vi "Teleop.vi"(10 "Match Info":T1={"Autonomous Elapsed Seconds"=0.0, "TeleOp Elapsed Seconds"=0.0, "Disabled Elapsed Seconds"=0.0, "Visited Autonomous"=FALSE, "Visited TeleOp"=FALSE, "Visited Disabled"=FALSE, "Autonomous Settings"={"Autonomous Style"=enum."Independent", "VI Refnum"=refnum}}, 11 "Call Context":T2) -> ()   [LabVIEW 2012]
doc: "This VI is called for each TeleOp packet received from the DS where the robot is not disabled. It is often used to read from the joysticks and update I/O or to update setpoints for timed control loops. It should complete and return within 20 milliseconds or it may miss DS packets."
uses:
  <vilib>/Rock Robotics/WPI/DriverStation/WPI_DriverStationDerivedRobotMode.ctl
  <vilib>/Rock Robotics/WPI/DriverStation/WPI_DriverStationMatch Info.ctl
  Robot Global Data.vi
  BotStatus.vi
  <vilib>/Rock Robotics/WPI/Joystick/WPI_JoystickGetSetRefNum.vi
  <vilib>/Rock Robotics/WPI/RobotDrive/WPI_RobotDriveGetSetRefNum.vi
panel:
  out "Numeric 1":dbl(slide) scale=0.0..100.0
  out "Boolean 2":bool
  out "Boolean 1":bool
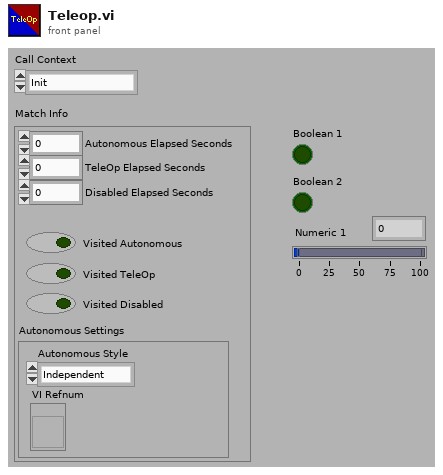
[diagram p1: front panel]
types:
  T1 = typedef "WPI_DriverStationMatch Info.ctl" = cluster{"Autonomous Elapsed Seconds":dbl, "TeleOp Elapsed Seconds":dbl, "Disabled Elapsed Seconds":dbl, "Visited Autonomous":bool, "Visited TeleOp":bool, "Visited Disabled":bool, "Autonomous Settings":cluster{"Autonomous Style":enum16{"Iterative", "Independent"}, "VI Refnum":refnum<vi>}}
  T2 = typedef "WPI_DriverStationDerivedRobotMode.ctl" = enum16{"Init", "Execute", "Stop"}
  T3 = typedef "WPI_JoystickDevRef.ctl" = cluster{"Device":T4}
  T4 = typedef "WPI_JoystickDeviceEnum.ctl" = enum16{"USB 1", "USB 2", "USB 3", "USB 4", "Kinect 1", "Kinect 2"}
  T5 = cluster{"Target Position X":dbl, "Target Position Y":dbl, "Target Found":bool}
  T6 = typedef "WPI_ServoDeviceRef.ctl" = cluster{"DeviceStatus":errorcluster, "Digital Module":T7, "PWM Channel":T8, "DeadBand":T9}
  T7 = typedef "FPGA_TypedefDigitalModule.ctl" = enum16{"Digital Module 1", "Digital Module 2"}
  T8 = typedef "FPGA_DIOPWMChannel.ctl" = enum8{"PWM 1", "PWM 2", "PWM 3", "PWM 4", "PWM 5", "PWM 6", "PWM 7", "PWM 8", "PWM 9", "PWM 10", "Invalid"}
  T9 = typedef "WPI_PWMDeadband.ctl" = cluster{"Name":string, "maxPositivePwm":i32, "minPositivePwm":i32, "centerPwm":i32, "maxNegativePwm":i32, "minNegativePwm":i32, "angularRange":u16}
  T10 = typedef "WPI_RobotDriveDevRef.ctl" = cluster{"DevStatus":errorcluster, "Motors[]":T11[], "Square Inputs":bool, "Max Output":dbl, "Isochronous":bool}
  T11 = typedef "WPI_MotorControlDeviceRef.ctl" = cluster{"DeviceStatus":errorcluster, "Type":enum16{"PWM", "CAN"}, "PWM":cluster{"Digital Module":T7, "PWM Channel":T8, "DeadBand":T9}, "CAN":cluster{"Device Number":u8, "Control Mode":T12, "Semaphore":T13, "Max Vout":dbl}, "Invert":bool, "TransformRef":T14, "InvTransformRef":T14}
  T12 = typedef "WPI_CANJaguar_ControlMode.ctl" = enum8{"Percent VBus", "Current", "Speed", "Position", "Voltage"}
  T13 = typedef "Semaphore RefNum" = refnum<k1>
  T14 = typedef "WPI_PWMTransform_ConPane.ctl" = refnum<vi>
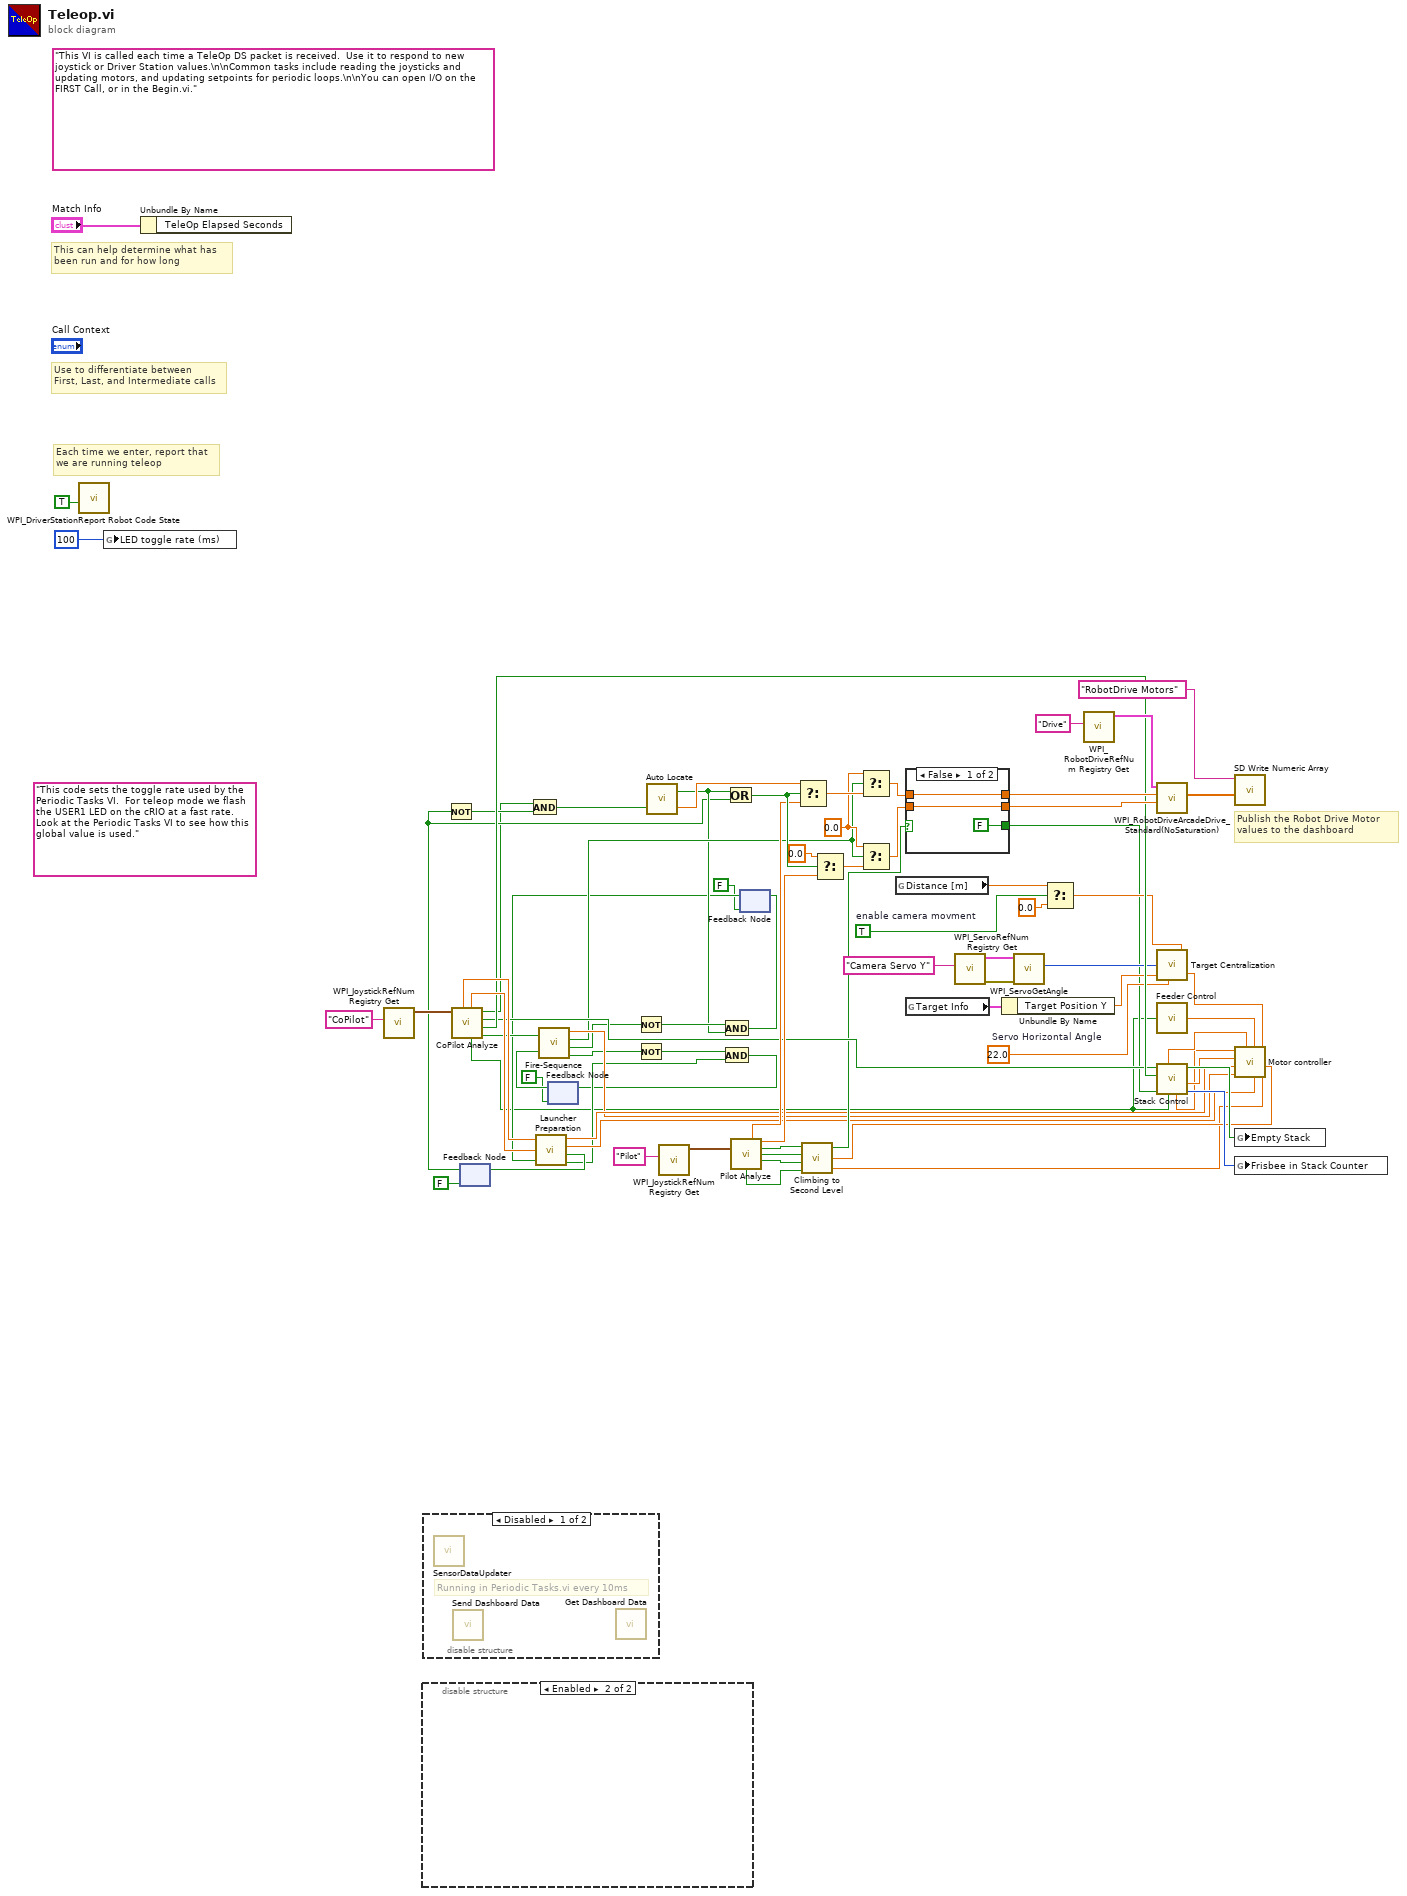
[diagram p0: block diagram]
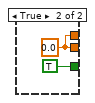
[diagram p3: hidden frame]
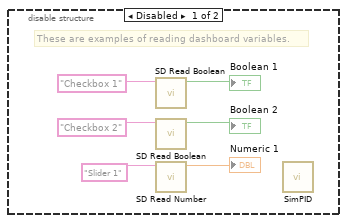
[diagram p4: hidden frame]
diagram:
  w32 = 22.0  # Servo Horizontal Angle
  w38 = TRUE  # enable camera movment
  w59 = 0.0
  (unwired) "This code sets the toggle rate used by the Periodic Tasks VI.  For teleop mode we flash the USER1 LED on the cRIO at a fast rate.  Look at the Periodic Tasks VI to see how this global value is used."
  (unwired) "This VI is called each time a TeleOp DS packet is received.  Use it to respond to new joystick or Driver Station values.\n\nCommon tasks include reading the joysticks and updating motors, and updating setpoints for periodic loops.\n\nYou can open I/O on the FIRST Call, or in the Begin.vi."
  # "Publish the Robot Drive Motor\nvalues to the dashboard"
  # "Each time we enter, report that\nwe are running teleop"
  # "Use to differentiate between\nFirst, Last, and Intermediate calls"
  # "This can help determine what has\nbeen run and for how long"
  n1 = call <vilib>:"WPI_DriverStationReport Robot Code State.vi"("TeleOp"=TRUE ("Autonomous")) -> ()  [unwired: 10 in, 1 out]
  n2 = global write "Robot Global Data.vi" "LED toggle rate (ms)"(u32 100 ("LED ms toggle rate")) -> ()
  n3 = Unbundle By Name("Match Info") -> ()  [unwired: 1 out]
  n4 = call <vilib>:"WPI_JoystickRefNum Registry Get.vi"("refnum name"="CoPilot") -> ("JoystickDevRef"=w67:T3)  [unwired: 1 in, 9 out]
  n5 = disable-structure shown="Enabled" {
    frame Disabled {
      # "These are examples of reading dashboard variables."
      n6 = call <vilib>:"SD Read Boolean.vi"("Name"="Checkbox 1" ("refnum name")) -> ("Boolean"=→"Boolean 1":bool)  [unwired: 8 in, 2 out]
      n7 = call <vilib>:"SD Read Boolean.vi"("Name"="Checkbox 2" ("refnum name")) -> ("Boolean"=→"Boolean 2":bool)  [unwired: 8 in, 2 out]
      n8 = call <vilib>:"SD Read Number.vi"("Name"="Slider 1" ("refnum name")) -> ("Numeric"=→"Numeric 1":dbl)  [unwired: 8 in, 2 out]
      n9 = call "SimPID.vi"() -> ()  [unwired: 9 in, 2 out]
    }
    frame Enabled {
    }
  }
  n10 = disable-structure shown="Disabled" {
    frame Disabled {
      # "Running in Periodic Tasks.vi every 10ms"
      n11 = call "SensorDataUpdater.vi"() -> ()  [unwired: 12 in]
      n12 = call "Send Dashboard Data.vi"() -> ()  [unwired: 12 in]
      n13 = call "Get Dashboard Data.vi"() -> ()  [unwired: 12 in]
    }
    frame Enabled {
    }
  }
  n14 = call "CoPilot Analyze.vi"("JoystickDevRef"=w67) -> ("La Fire at will?"=w57:bool, "Ejection"=w50:bool, "Suction"=w49:bool, "Aim?"=w3:bool, "Feeder?"=w1:bool, "Elevation"=w58:dbl, "Shoot Motors"=w66:dbl)  [unwired: 4 in]
  n15 = feedback #1(FALSE ("Aim?")) -> (w4:bool)
  n16 = Not(x=w4) -> (.not. x?=w5:bool)
  n17 = And(x=w3, y=w5) -> (x .and. y?=w2:bool)
  n18 = feedback #2(FALSE) -> (w7:bool)
  n19 = call "Fire-Sequence.vi"("La Fire at will?"=w57, "Ready?"=w7) -> ("Transfer"=w23:dbl, "Fire!"=w21:bool, "Set?"=w16:bool, "Ready?"=w10:bool)
  n20 = Not(x=w16) -> (.not. x?=w17:bool)
  n21 = Not(x=w10) -> (.not. x?=w11:bool)
  n22 = call "Auto Locate.vi"("Aim?"=w2) -> ("X Drive Arcade"=w56:dbl, "Set?"=w15:bool)  [unwired: 1 in]
  n23 = call <vilib>:"WPI_JoystickRefNum Registry Get.vi"("refnum name"="Pilot") -> ("JoystickDevRef"=w69:T3)  [unwired: 1 in, 9 out]
  n24 = And(x=w17, y=w15) -> (x .and. y?=w14:bool)
  n25 = Or(x=w15, y=w4) -> (x .or. y?=w65:bool)
  n26 = call "Pilot Analyze.vi"("JoystickDevRef"=w69) -> ("x"=w64:dbl, "y"=w63:dbl, "close arms"=w47:bool, "second preperation"=w46:bool, "pull wire"=w45:bool, "open arms"=w44:bool)  [unwired: 7 in, 2 out]
  n27 = feedback-in #3(w14) -> ()
  n28 = feedback #3(FALSE) -> (w13:bool)
  n29 = call "Launcher Preparation.vi"("Shooting Motors"=w66, "Elevation"=w58, "Set?"=w13) -> ("Cannon"=w28:dbl, "zAvit"=w20:dbl, "Aim?"=w18:bool, "Ready?"=w9:bool)
  n30 = feedback-in #1(w18) -> ()
  n31 = And(x=w11, y=w9) -> (x .and. y?=w8:bool)
  n32 = feedback-in #2(w8) -> ()
  n33 = Select(t=w56, s=w65, f=w64) -> (s? t:f=w61:dbl)
  n34 = call "Climbing to Second Level.vi"("Open arms"=w44, "pull wire"=w45, "Second Preperation"=w46, "close arms"=w47) -> ("Telescopic Arms"=w29:dbl, "Canenet"=w30:dbl, "Prep 2"=w48:bool)
  n35 = Select(t=0.0, s=w65, f=w63) -> (s? t:f=w60:dbl)
  n36 = Select(t=w59, s=w21, f=w61) -> (s? t:f=w55:dbl)
  n37 = Select(t=w59, s=w21, f=w60) -> (s? t:f=w54:dbl)
  n38 = global read "BotStatus.vi" "Distance [m]"() -> (w37:dbl)
  n39 = case shown="False" w48 {
    tunnel: w55 -> [w85 _]
    tunnel: w54 -> [w86 _]
    tunnel: [w85 w88] -> w53
    tunnel: [w86 w88] -> w52
    tunnel: [FALSE TRUE ("Disable Stack")] -> w22
    frame False {
    }
    frame True {
      w88 = 0.0 ("x")
    }
  }
  n40 = global read "BotStatus.vi" "Target Info"() -> (w43:T5)
  n41 = call <vilib>:"WPI_ServoRefNum Registry Get.vi"("refnum name"="Camera Servo Y") -> ("error out"=w42:errorcluster, "ServoDeviceRef"=w41:T6)  [unwired: 9 in]
  n42 = Unbundle By Name(w43) -> ("Target Position Y"=w34:dbl)
  n43 = call <vilib>:"WPI_ServoGetAngle.vi"("ServoDeviceRef"=w41, "error in (no error)"=w42) -> ("Angle"=w39:u16)  [unwired: 6 in, 2 out]
  n44 = Select(t=w37, s=w38, f=0.0) -> (s? t:f=w35:dbl)
  n45 = call <vilib>:"WPI_RobotDriveRefNum Registry Get.vi"("refnum name"="Drive") -> ("RobotDriveDevRef"=w75:T10)  [unwired: 1 in, 9 out]
  n46 = call <vilib>:"WPI_RobotDriveArcadeDrive_Standard(NoSaturation).vi"("Y axis value"=w52, "X axis value"=w53, "RobotDriveDevRef"=w75) -> ("Motor Values"=w70:dbl[])  [unwired: 1 in, 7 out]
  n47 = call "Target Centralization.vi"("Servo Angle in"=w39, "Camera Axis Position"=w34, "Servo Horizontal Angle"=w32, "Distance From Target"=w35) -> ("Servo Angle out"=w31:dbl)  [unwired: 2 in]
  n48 = call "Feeder Control.vi"("Collect from Feeder?"=w1) -> ("Feeder"=w27:dbl)
  n49 = call "Stack Control.vi"("Feeder Mode Enabled"=w1, "Disable Stack"=w22, "Eject"=w50, "Suck"=w49) -> ("frisbee counter"=w33:i16, "Roller"=w25:dbl, "Empty Stack"=w51:bool, "Conveyer Belt"=w24:dbl, "Flipper"=w26:dbl)  [unwired: 1 in, 2 out]
  n50 = call <vilib>:"SD Write Numeric Array.vi"("Numeric Array"=w70, "Name"="RobotDrive Motors") -> ()  [unwired: 8 in, 2 out]
  n51 = call "Motor controller.vi"("Conveyer Belt"=w24, "Roller"=w25, "Cannon"=w28, "Transfer"=w23, "Flipper"=w26, "Feeder"=w27, "zAvit"=w20, "Camera Servo Y"=w31, "Canenet"=w30, "Climb Telescopic"=w29) -> ()  [unwired: 1 in]
  n52 = global write "BotStatus.vi" "Empty Stack"(w51) -> ()
  n53 = global write "BotStatus.vi" "Frisbee in Stack Counter"(w33) -> ()
